vi "一体站流程自动启动.vi"(11 "参数":T1={"CODCr"={"启动测量模式"={"测量模式"=enum."水样测量"}, "确定按钮"=TRUE}, "参数启用"={"多参数"=FALSE, "CODMn"=FALSE, "总磷"=FALSE, "总氮"=FALSE, "氨氮"=FALSE, "CODcr"=FALSE}}) -> ()   [LabVIEW 2016, in "PLC.lvlib"]
uses:
  PLC.lvlib
  API/CodCr/CodCr.lvlib
panel:
  out "枚举":enum16{"初始化", "采配水启动", "等待", "配水", "排水", "结束"}(ring)
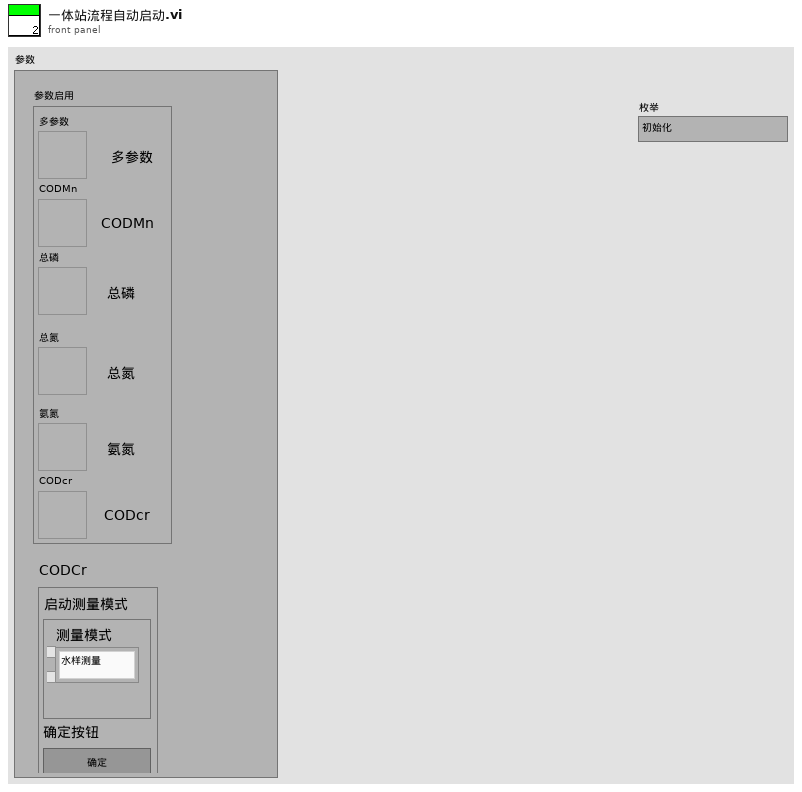
[diagram p1: front panel]
types:
  T1 = cluster{"CODCr":cluster{"启动测量模式":cluster{"测量模式":enum16{"水样测量", "标样核查", "零点核查", "跨度核查", "空白测试", "加标回收", "平行样", "校零", "校标"}}, "确定按钮":bool}, "参数启用":cluster{"多参数":bool, "CODMn":bool, "总磷":bool, "总氮":bool, "氨氮":bool, "CODcr":bool}}
  T2 = cluster{"命令":string, cluster{"starting address":u16, "holding register value":u16}}
  T3 = enum16{"待机", "启动氨氮", "氨氮测量中", "启动总磷", "总磷测量中", "结束"}
  T4 = cluster{"站号 2":u16, "量程切换":enum32{"H", "L", "AUTO"}, "控制命令":enum16{"启动测量", "标样核查", "零点核查", "跨度核查", "空白测试", "平行样测试", "加标回收", "空白校准", "标样校准", "初始化（清洗）", "停止测试", "仪器重启", "校时", "模式设置", "测量间隔设置"}, "模式设置":enum16{"待机", "连续模式", "周期模式", "定点模式", "受控模式", "手动模式"}, "测量间隔":u16}
  T5 = cluster{"测量模式":enum16{"水样测量", "标样核查", "零点核查", "跨度核查", "空白测试", "加标回收", "平行样", "校零", "校标"}}
  T6 = cluster{"时间标识":timestamp, "设备":string, "日志信息":string, "流程参数":string}
  T7 = cluster{"时间标识":timestamp, "设备":string, "日志信息":string}
  T8 = enum16{"空闲", "水样测试", "标样核查", "零点核查", "跨度核查", "空白测试", "平行样测试", "加标回收", "空白校准", "标样校准", "初始化（清洗）"}
  T9 = cluster{"R0":i16, "R1":i16, "R2":i16, "R3":i16, "R4":i16, "R5":i16, "R6":i16, "R7":i16, "R8":i16, "R9":i16, "R10":i16, "R11":i16, "R12":i16, "R13":i16, "R14":i16, "R15":i16, "R16":i16, "R17":i16, "R18":i16, "R19":i16, "R20":i16, "R21":i16, "R22":i16, "R23":i16, "R24":i16, "R25":i16, "R26":i16, "R27":i16, "R28":i16, "R29":i16, "R30":i16, "R31":i16, "R32":i16, "R33":i16, "R34":i16, "R35":i16, "R36":i16, "R37":i16, "R38":i16, "R39":i16, "R40":i16, "R41":i16, "R42":i16, "R43":i16, "R44":i16, "R45":i16, "R46":i16, "R47":i16, "R48":i16, "R49":i16, "R50":i16, "R51":i16, "R52":i16, "R53":i16, "R54":i16, "R55":i16, "R56":i16}
  T10 = enum32{"Bad", "Idle", "Run top level", "Running"}
  T11 = cluster{"水样测试量程模式":enum16{"H", "L", "AUTO"}, "空白核查量程模式":enum16{"H", "L", "AUTO"}, "跨度核查量程模式":enum16{"H", "L", "AUTO"}}
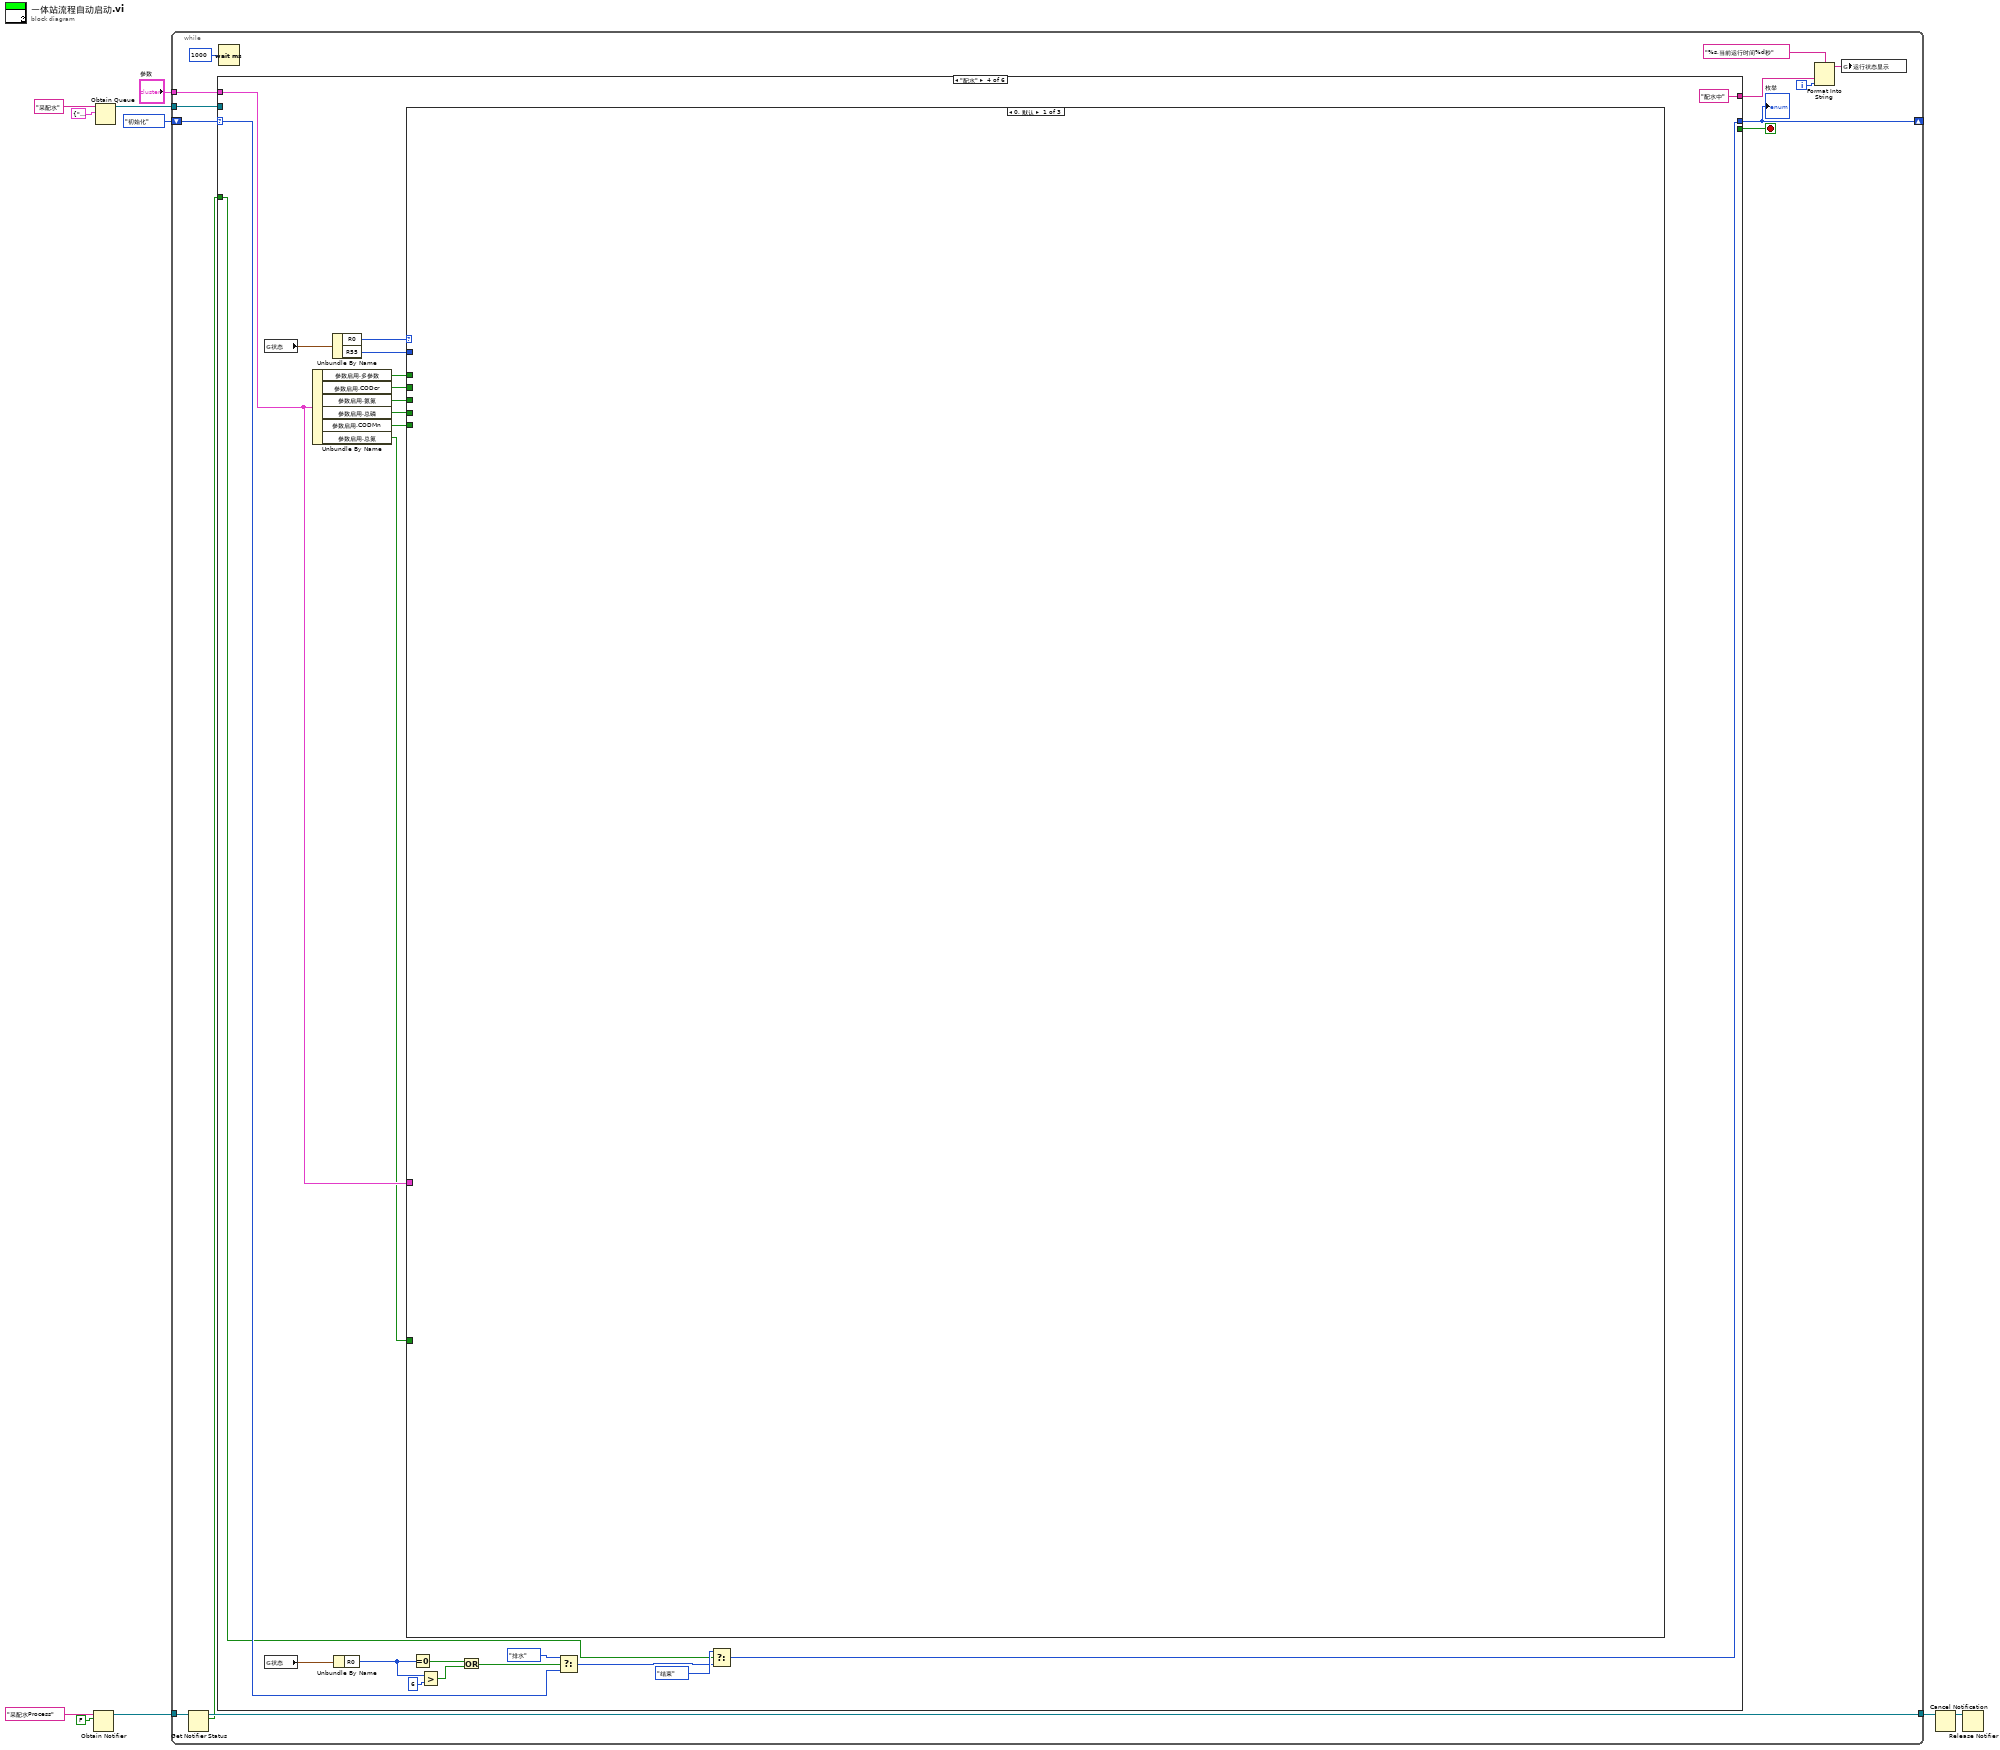
[diagram p0: block diagram]
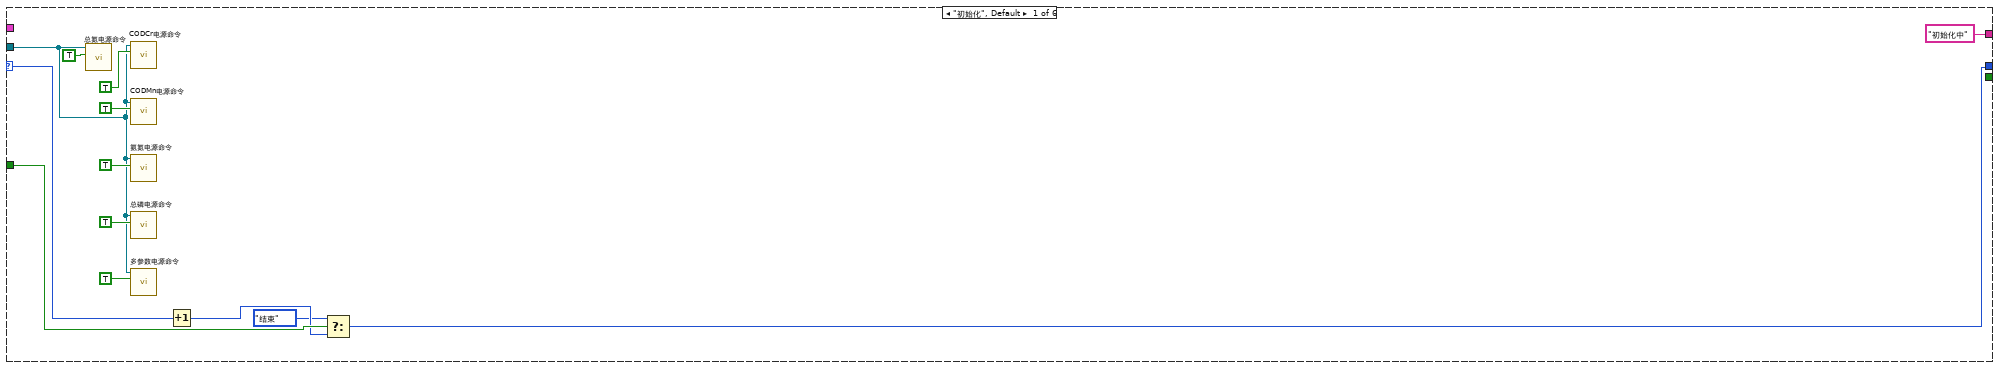
[diagram p2: hidden frame]
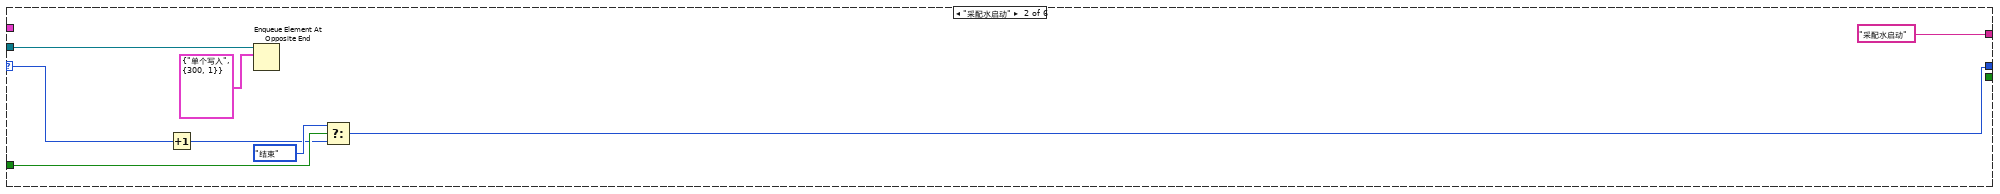
[diagram p3: hidden frame]
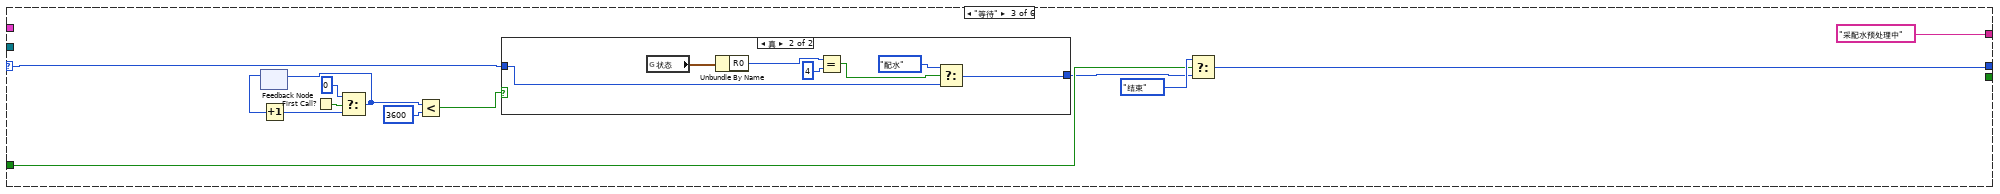
[diagram p4: hidden frame]
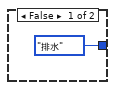
[diagram p5: hidden frame]
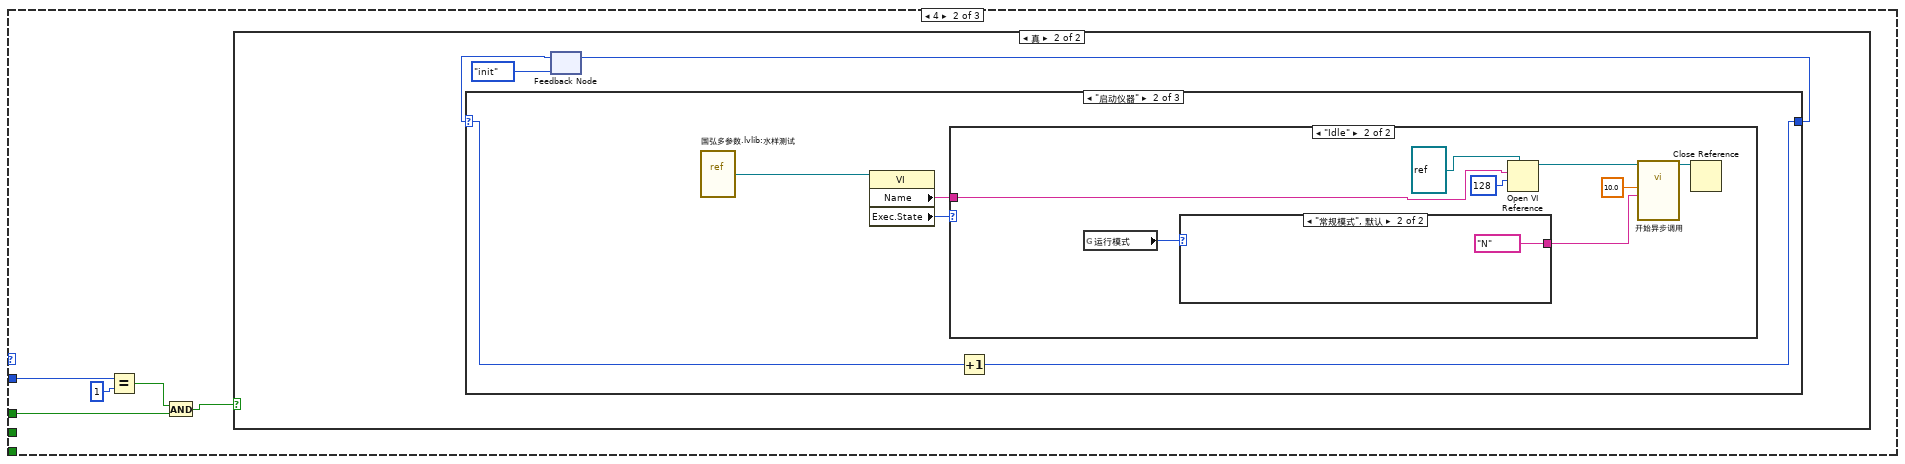
[diagram p6: hidden frame]
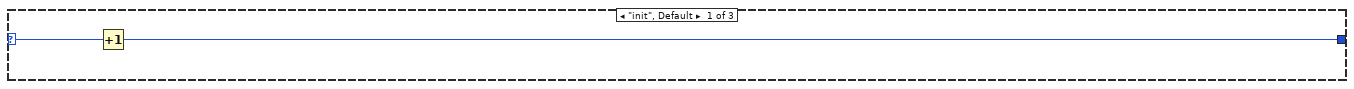
[diagram p8: hidden frame]
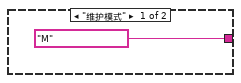
[diagram p10: hidden frame]
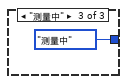
[diagram p11: hidden frame]
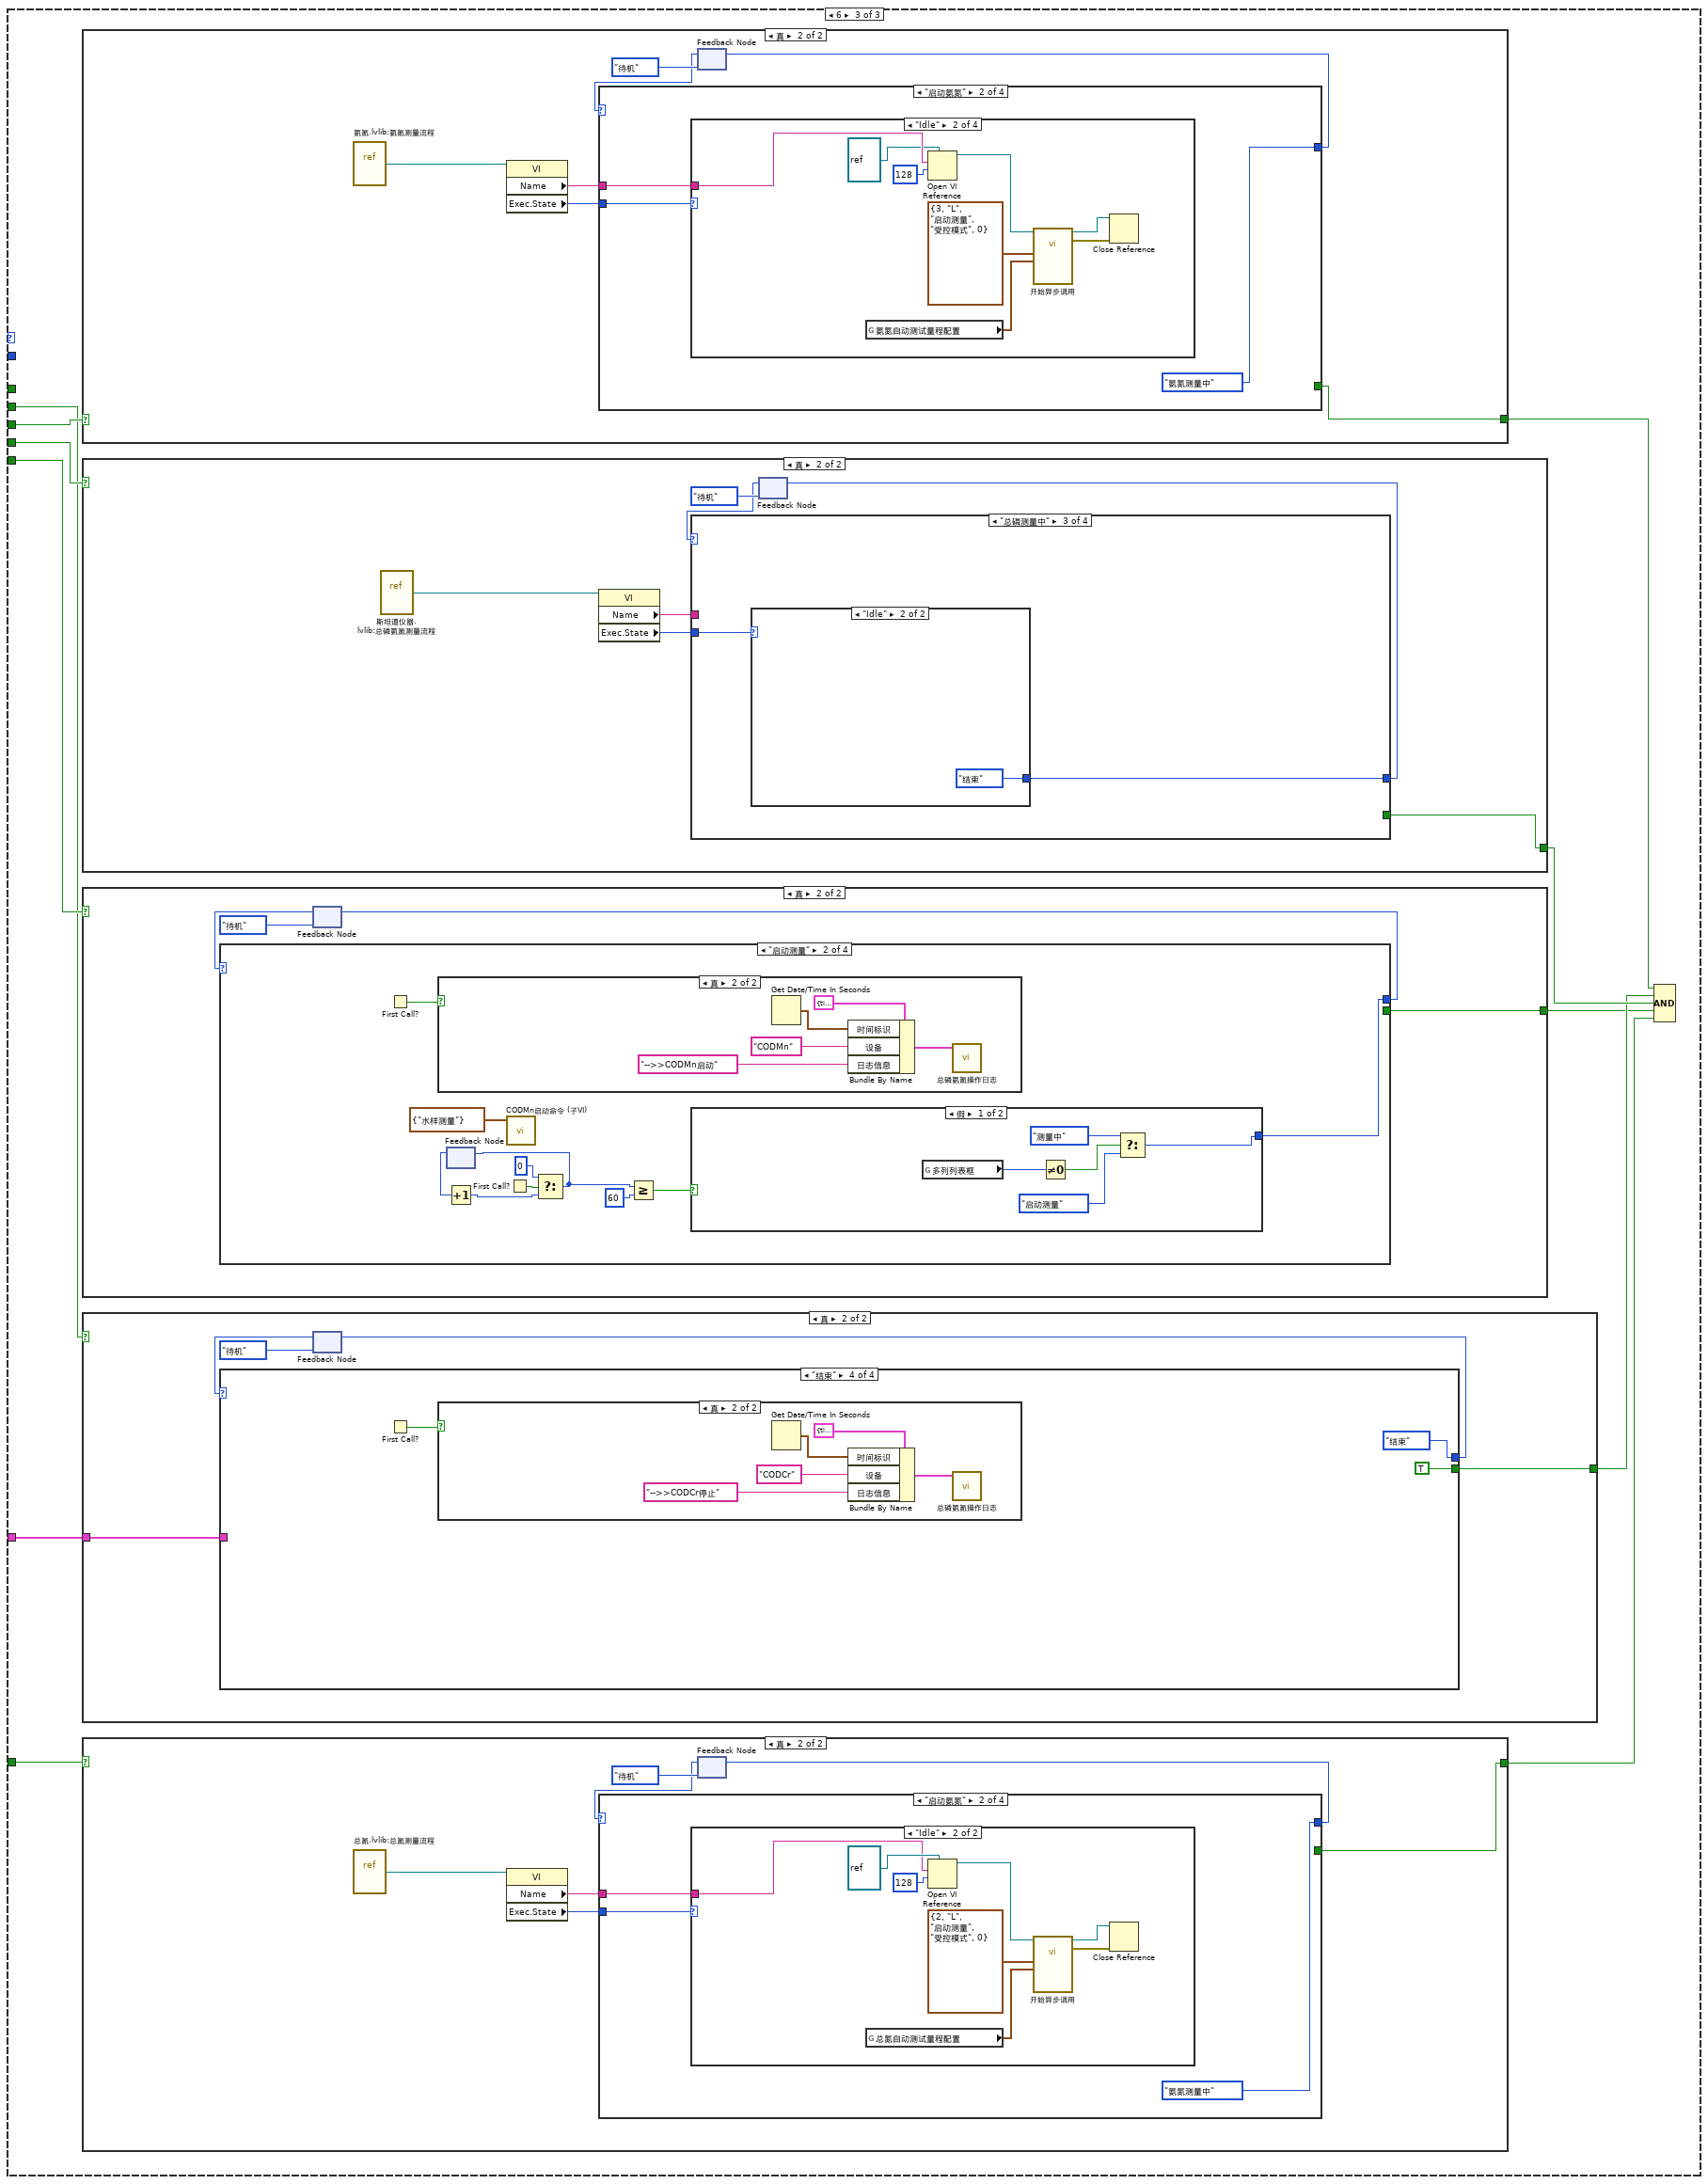
[diagram p12: hidden frame]
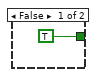
[diagram p13: hidden frame]
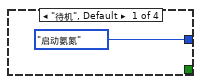
[diagram p14: hidden frame]
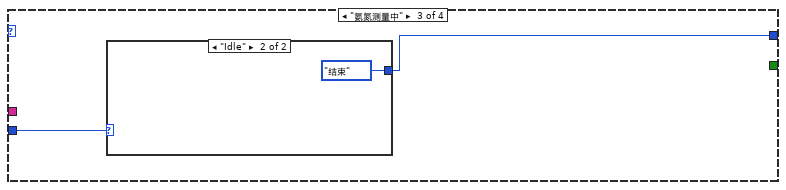
[diagram p16: hidden frame]
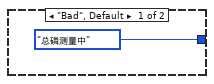
[diagram p17: hidden frame]
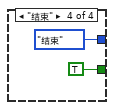
[diagram p18: hidden frame]
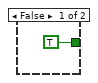
[diagram p19: hidden frame]
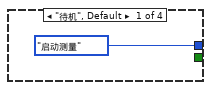
[diagram p20: hidden frame]
diagram:
  n1 = Obtain Notifier(name (unnamed)="采配水Process" ("名称（未命名）"), notification data type=FALSE) -> (notifier out=w3:refnum<notifier>)  [unwired: 2 in, 2 out]
  n2 = Obtain Queue(name (unnamed)="采配水" ("名称（未命名）"), element data type=cluster{"命令":string, "数据":variant} {"命令"="", "数据"=variant}) -> (queue out=w8:refnum<queue>)  [unwired: 3 in, 2 out]
  n3 = while {
    tunnel: w8 -> [w23]
    shift-right: [w21] -> _
    shift-left: enum16{"初始化", "采配水启动", "等待", "配水", "排水", "结束"}."初始化" ("枚举") -> [w22]
    tunnel: "参数" -> [w19]
    tunnel: w3 -> [w18]
    tunnel: [w17] -> w2
    i -> [w14]
    stop <- w13 stop-if-true
    n4 = Get Notifier Status(notifier=w18) -> (notifier out=w17:refnum<notifier>, current notification=w12:bool)  [unwired: 1 in, 3 out]
    n5 = case shown="\"配水\"" w22 {
      selector: w22 -> [w36 w42 w55 w87 w306 w312]
      tunnel: w23 -> [w25 w43 _ _ w307 _]
      tunnel: [w32 w37 w45 w83 w301 w311] -> w21
      tunnel: [_ _ _ _ _ TRUE] -> w13
      tunnel: w19 -> [_ _ _ w79 _ _]
      tunnel: ["初始化中" ("输入 1") "采配水启动" ("输入 1") "采配水预处理中" ("输入 1") "配水中" ("输入 1") "排水中" ("输入 1") "结束" ("输入 1")] -> w15
      tunnel: w12 -> [w34 w39 w47 w85 w303 _]
      frame "初始化", Default {
        n6 = call "总氮电源命令.vi"("通电/断电"=TRUE, "队列"=w25) -> ()  [unwired: 9 in, 1 out]
        n7 = call "CODCr电源命令.vi"("通电/断电"=TRUE, "队列"=w25) -> ()  [unwired: 9 in, 1 out]
        n8 = call "CODMn电源命令.vi"("通电/断电"=TRUE, "队列"=w25) -> ()  [unwired: 9 in, 1 out]
        n9 = call "氨氮电源命令.vi"("通电/断电"=TRUE, "队列"=w25) -> ()  [unwired: 9 in, 1 out]
        n10 = call "总磷电源命令.vi"("通电/断电"=TRUE, "队列"=w25) -> ()  [unwired: 9 in, 1 out]
        n11 = call "多参数电源命令.vi"("通电/断电"=TRUE, "队列"=w25) -> ()  [unwired: 9 in, 1 out]
        n12 = Increment(x=w36) -> (x+1=w33:enum16{"初始化", "采配水启动", "等待", "配水", "排水", "结束"})
        n13 = Select(t=enum16{"初始化", "采配水启动", "等待", "配水", "排水", "结束"}."结束", s=w34, f=w33) -> (s? t:f=w32:enum16{"初始化", "采配水启动", "等待", "配水", "排水", "结束"})
      }
      frame "采配水启动" {
        n14 = Increment(x=w42) -> (x+1=w38:enum16{"初始化", "采配水启动", "等待", "配水", "排水", "结束"})
        n15 = Enqueue Element At Opposite End(queue=w43, element=T2 {"命令"="单个写入", {"starting address"=300, "holding register value"=1}} ("元素")) -> ()  [unwired: 2 in, 3 out]
        n16 = Select(t=enum16{"初始化", "采配水启动", "等待", "配水", "排水", "结束"}."结束", s=w39, f=w38) -> (s? t:f=w37:enum16{"初始化", "采配水启动", "等待", "配水", "排水", "结束"})
      }
      frame "等待" {
        n17 = feedback #1() -> (w52:i32)  [unwired: 1 in]
        n18 = Increment(x=w52) -> (x+1=w51:i32)
        n19 = First Call?() -> (First Call?: T/F=w53:bool)
        n20 = Select(t=0, s=w53, f=w51) -> (s? t:f=w50:i32)
        n21 = feedback-in #1(w50) -> ()
        n22 = Less?(x=w50, y=3600) -> (x < y?=w56:bool)
        n23 = case shown="真" w56 {
          tunnel: w55 -> [_ w60]
          tunnel: [enum16{"初始化", "采配水启动", "等待", "配水", "排水", "结束"}."排水" ("枚举") w59] -> w46
          frame False {
          }
          frame True {
            n24 = global read "采配水全局变量.vi" "状态"() -> (w65:T9)
            n25 = Unbundle By Name(w65) -> ("R0"=w64:i16)
            n26 = Equal?(x=w64, y=i16 4) -> (x = y?=w62:bool)
            n27 = Select(t=enum16{"初始化", "采配水启动", "等待", "配水", "排水", "结束"}."配水" ("枚举"), s=w62, f=w60) -> (s? t:f=w59:enum16{"初始化", "采配水启动", "等待", "配水", "排水", "结束"})
          }
        }
        n28 = Select(t=enum16{"初始化", "采配水启动", "等待", "配水", "排水", "结束"}."结束", s=w47, f=w46) -> (s? t:f=w45:enum16{"初始化", "采配水启动", "等待", "配水", "排水", "结束"})
      }
      frame "配水" {
        n29 = global read "采配水全局变量.vi" "状态"() -> (w70:T9)
        n30 = global read "采配水全局变量.vi" "状态"() -> (w77:T9)
        n31 = Unbundle By Name(w79) -> ("参数启用.多参数"=w68:bool, "参数启用.CODcr"=w78:bool, "参数启用.氨氮"=w82:bool, "参数启用.总磷"=w81:bool, "参数启用.CODMn"=w80:bool, "参数启用.总氮"=w71:bool)
        n32 = Unbundle By Name(w70) -> ("R0"=w69:i16, "R55"=w66:i16)
        n33 = Unbundle By Name(w77) -> ("R0"=w76:i16)
        n34 = case shown="0, 默认" w69 {
          tunnel: w82 -> [_ _ w125]
          tunnel: w81 -> [_ _ w124]
          tunnel: w80 -> [_ _ w121]
          tunnel: w79 -> [_ _ w120]
          tunnel: w78 -> [_ _ w119]
          tunnel: w71 -> [_ _ w116]
          tunnel: w68 -> [_ w90 _]
          tunnel: w66 -> [_ w93 _]
          frame 0, Default {
          }
          frame 4 {
            n35 = Equal?(x=w93, y=i16 1) -> (x = y?=w91:bool)
            n36 = And(x=w91, y=w90) -> (x .and. y?=w89:bool)
            n37 = case shown="真" w89 {
              frame False {
              }
              frame True {
                n38 = feedback #2(enum16{"init", "启动仪器", "测量中"}."init") -> (w95:enum16{"init", "启动仪器", "测量中"})
                n39 = case shown="\"启动仪器\"" w95 {
                  selector: w95 -> [w98 w103 _]
                  tunnel: [w97 w102 enum16{"init", "启动仪器", "测量中"}."测量中"] -> w96
                  frame "init", Default {
                    n40 = Increment(x=w98) -> (x+1=w97:enum16{"init", "启动仪器", "测量中"})
                  }
                  frame "启动仪器" {
                    n41 = vi-ref "国弘多参数.lvlib:水样测试.vi"() -> (w100:refnum<vi>)
                    n42 = property class="VI"(reference=w100) -> ("Name"=w99:string, "Exec.State"=w101:T10)  [unwired: 1 in, 2 out]
                    n43 = case shown="\"Idle\"" w101 {
                      tunnel: w99 -> [_ w110]
                      frame "Bad", Default {
                      }
                      frame "Idle" {
                        n44 = global read "系统变量.vi" "运行模式"() -> (w107:enum16{"维护模式", "常规模式", "应急模式", "质控模式"})
                        n45 = case shown="\"常规模式\", 默认" w107 {
                          tunnel: ["M" ("数据标记表") "N" ("数据标记表")] -> w105
                          frame "维护模式" {
                          }
                          frame "常规模式", Default {
                          }
                        }
                        n46 = Open VI Reference(type specifier VI Refnum (for type only)=refnum<vi> refnum, vi path=w110, options=128 ("选项")) -> (vi reference=w109:refnum<vi>)  [unwired: 3 in, 1 out]
                        n47 = call-by-ref "开始异步调用"(reference=w109, "数据标记表"=w105, "水样测试时间"=10.0) -> (reference out=w108:refnum<vi>)  [unwired: 11 in, 1 out]
                        n48 = Close Reference(reference=w108) -> ()  [unwired: 1 in, 1 out]
                      }
                    }
                    n49 = Increment(x=w103) -> (x+1=w102:enum16{"init", "启动仪器", "测量中"})
                  }
                  frame "测量中" {
                  }
                }
                n50 = feedback-in #2(w96) -> ()
              }
            }
          }
          frame 6 {
            n51 = case shown="真" w125 {
              tunnel: [TRUE w279] -> w123
              frame False {
              }
              frame True {
                n52 = vi-ref "氨氮.lvlib:氨氮测量流程.vi"() -> (w278:refnum<vi>)
                n53 = property class="VI"(reference=w278) -> ("Name"=w277:string, "Exec.State"=w276:T10)  [unwired: 1 in, 2 out]
                n54 = feedback #3(T3."待机") -> (w281:T3)
                n55 = case shown="\"启动氨氮\"" w281 {
                  tunnel: [T3."启动氨氮" T3."氨氮测量中" w295 T3."结束"] -> w280
                  tunnel: [_ _ _ TRUE] -> w279
                  tunnel: w277 -> [_ w285 _ _]
                  tunnel: w276 -> [_ w284 w296 _]
                  frame "待机", Default {
                  }
                  frame "启动氨氮" {
                    n56 = case shown="\"Idle\"" w284 {
                      tunnel: w285 -> [_ w291 _ _]
                      frame "Bad", Default {
                      }
                      frame "Idle" {
                        n57 = global read "系统设置全局变量.vi" "氨氮自动测试量程配置"() -> (w288:T11)
                        n58 = Open VI Reference(type specifier VI Refnum (for type only)=refnum<vi> refnum, vi path=w291, options=128 ("选项")) -> (vi reference=w292:refnum<vi>)  [unwired: 3 in, 1 out]
                        n59 = call-by-ref "开始异步调用"(reference=w292, "量程模式"=w288, "参数"=T4 {"站号 2"=3, "量程切换"=enum."L", "控制命令"=enum."启动测量", "模式设置"=enum."受控模式", "测量间隔"=0}) -> (reference out=w293:refnum<vi>, error out=w294:errorcluster)  [unwired: 11 in]
                        n60 = Close Reference(reference=w293, error in (no error)=w294) -> ()  [unwired: 1 out]
                      }
                      frame "Run top level" {
                      }
                      frame "Running" {
                      }
                    }
                  }
                  frame "氨氮测量中" {
                    n61 = case shown="\"Bad\", 默认" w296 {
                      tunnel: [T3."氨氮测量中" T3."结束"] -> w295
                      frame "Bad", Default {
                      }
                      frame "Idle" {
                      }
                    }
                  }
                  frame "结束" {
                  }
                }
                n62 = feedback-in #3(w280) -> ()
              }
            }
            n63 = case shown="真" w124 {
              tunnel: [TRUE w253] -> w122
              frame False {
              }
              frame True {
                n64 = vi-ref "斯坦道仪器.lvlib:总磷氨氮测量流程.vi"() -> (w252:refnum<vi>)
                n65 = property class="VI"(reference=w252) -> ("Name"=w251:string, "Exec.State"=w250:T10)  [unwired: 1 in, 2 out]
                n66 = feedback #4(T3."待机") -> (w255:T3)
                n67 = case shown="\"总磷测量中\"" w255 {
                  tunnel: [T3."启动总磷" T3."总磷测量中" w269 T3."结束"] -> w254
                  tunnel: [_ _ _ TRUE] -> w253
                  tunnel: w251 -> [_ w260 _ _]
                  tunnel: w250 -> [_ w259 w270 _]
                  frame "待机", Default {
                  }
                  frame "启动总磷" {
                    n68 = case shown="\"Idle\"" w259 {
                      tunnel: w260 -> [_ w267]
                      frame "Bad", Default {
                      }
                      frame "Idle" {
                        n69 = global read "系统设置全局变量.vi" "总磷自动测试量程配置"() -> (w262:T11)
                        n70 = Open VI Reference(type specifier VI Refnum (for type only)=refnum<vi> refnum, vi path=w267, options=128 ("选项")) -> (vi reference=w266:refnum<vi>)  [unwired: 3 in, 1 out]
                        n71 = call-by-ref "开始异步调用"(reference=w266, "量程模式"=w262, "参数"=T4 {"站号 2"=1, "量程切换"=enum."L", "控制命令"=enum."启动测量", "模式设置"=enum."受控模式", "测量间隔"=0}) -> (reference out=w265:refnum<vi>, error out=w264:errorcluster)  [unwired: 11 in]
                        n72 = Close Reference(reference=w265, error in (no error)=w264) -> ()  [unwired: 1 out]
                      }
                    }
                  }
                  frame "总磷测量中" {
                    n73 = case shown="\"Idle\"" w270 {
                      tunnel: [T3."总磷测量中" T3."结束"] -> w269
                      frame "Bad", Default {
                      }
                      frame "Idle" {
                      }
                    }
                  }
                  frame "结束" {
                  }
                }
                n74 = feedback-in #4(w254) -> ()
              }
            }
            n75 = case shown="真" w121 {
              tunnel: [TRUE w153] -> w117
              frame False {
              }
              frame True {
                n76 = feedback #5(enum16{"待机", "启动测量", "测量中", "结束"}."待机") -> (w155:enum16{"待机", "启动测量", "测量中", "结束"})
                n77 = case shown="\"启动测量\"" w155 {
                  tunnel: [enum16{"待机", "启动测量", "测量中", "结束"}."启动测量" w167 w186 enum16{"待机", "启动测量", "测量中", "结束"}."结束"] -> w154
                  tunnel: [_ _ _ TRUE] -> w153
                  frame "待机", Default {
                  }
                  frame "启动测量" {
                    n78 = First Call?() -> (First Call?: T/F=w158:bool)
                    n79 = case shown="真" w158 {
                      frame False {
                      }
                      frame True {
                        n80 = Get Date/Time In Seconds() -> (seconds since 1Jan1904=w172:timestamp)
                        n81 = Bundle By Name(cluster=T6 {"时间标识"=timestamp(0 s since 1904-01-01), "设备"="", "日志信息"="", "流程参数"=""} ("data in"), "时间标识"=w172, "设备"="CODMn", "日志信息"="-->>CODMn启动") -> (w168:T6)
                        n82 = call "总磷氨氮操作日志.vi"("data in"=w168) -> ()  [unwired: 11 in]
                      }
                    }
                    n83 = feedback #6() -> (w163:i32)  [unwired: 1 in]
                    n84 = Increment(x=w163) -> (x+1=w164:i32)
                    n85 = First Call?() -> (First Call?: T/F=w162:bool)
                    n86 = call "CODMn启动命令 (子VI).vi"("启动测量模式"=T5 {"测量模式"=enum."水样测量"}) -> ()  [unwired: 11 in]
                    n87 = Select(t=0, s=w162, f=w164) -> (s? t:f=w165:i32)
                    n88 = feedback-in #6(w165) -> ()
                    n89 = Greater Or Equal?(x=w165, y=60) -> (x >= y?=w160:bool)
                    n90 = case shown="假" w160 {
                      tunnel: [w174 enum16{"待机", "启动测量", "测量中", "结束"}."结束"] -> w167
                      frame False {
                        n91 = global read "运行时序全局变量.vi" "多列列表框"() -> (w173:i32)
                        n92 = Not Equal To 0?(x=w173) -> (x != 0?=w175:bool)
                        n93 = Select(t=enum16{"待机", "启动测量", "测量中", "结束"}."测量中", s=w175, f=enum16{"待机", "启动测量", "测量中", "结束"}."启动测量") -> (s? t:f=w174:enum16{"待机", "启动测量", "测量中", "结束"})
                      }
                      frame True {
                        n94 = Get Date/Time In Seconds() -> (seconds since 1Jan1904=w178:timestamp)
                        n95 = Bundle By Name(cluster=T7 {"时间标识"=timestamp(0 s since 1904-01-01), "设备"="", "日志信息"=""} ("data in"), "时间标识"=w178, "设备"="CODMn", "日志信息"="CODMn启动失败") -> (w182:T7)
                        n96 = call "总磷氨氮报警信息.vi"("data in"=w182) -> ()  [unwired: 11 in]
                      }
                    }
                  }
                  frame "测量中" {
                    n97 = global read "运行时序全局变量.vi" "多列列表框"() -> (w185:i32)
                    n98 = Equal To 0?(x=w185) -> (x = 0?=w184:bool)
                    n99 = case shown="假" w184 {
                      tunnel: [w187 enum16{"待机", "启动测量", "测量中", "结束"}."结束"] -> w186
                      frame False {
                        n100 = flat-sequence {
                          tunnel: [enum16{"待机", "启动测量", "测量中", "结束"}."测量中"] -> w187
                          frame #0 {
                            n101 = Wait (ms)(milliseconds to wait=u32 1000 ("等待时间（毫秒）")) -> ()  [unwired: 1 out]
                          }
                          frame #1 {
                          }
                        }
                      }
                      frame True {
                      }
                    }
                  }
                  frame "结束" {
                    n102 = First Call?() -> (First Call?: T/F=w191:bool)
                    n103 = case shown="真" w191 {
                      frame False {
                      }
                      frame True {
                        n104 = Get Date/Time In Seconds() -> (seconds since 1Jan1904=w198:timestamp)
                        n105 = Bundle By Name(cluster=T6 {"时间标识"=timestamp(0 s since 1904-01-01), "设备"="", "日志信息"="", "流程参数"=""} ("data in"), "时间标识"=w198, "设备"="CODMn", "日志信息"="-->>CODMn停止") -> (w194:T6)
                        n106 = call "总磷氨氮操作日志.vi"("data in"=w194) -> ()  [unwired: 11 in]
                      }
                    }
                  }
                }
                n107 = feedback-in #5(w154) -> ()
              }
            }
            n108 = case shown="真" w119 {
              tunnel: [TRUE w201] -> w118
              tunnel: w120 -> [_ w200]
              frame False {
              }
              frame True {
                n109 = feedback #7(enum16{"待机", "启动测量", "测量中", "结束"}."待机") -> (w203:enum16{"待机", "启动测量", "测量中", "结束"})
                n110 = case shown="\"结束\"" w203 {
                  tunnel: [enum16{"待机", "启动测量", "测量中", "结束"}."启动测量" w215 w236 enum16{"待机", "启动测量", "测量中", "结束"}."结束"] -> w202
                  tunnel: w200 -> [_ w216 _ _]
                  tunnel: [_ _ _ TRUE] -> w201
                  frame "待机", Default {
                  }
                  frame "启动测量" {
                    n111 = Unbundle By Name(w216) -> ("CODCr.启动测量模式"=w214:T5)
                    n112 = First Call?() -> (First Call?: T/F=w206:bool)
                    n113 = case shown="真" w206 {
                      frame False {
                      }
                      frame True {
                        n114 = Get Date/Time In Seconds() -> (seconds since 1Jan1904=w221:timestamp)
                        n115 = Bundle By Name(cluster=T6 {"时间标识"=timestamp(0 s since 1904-01-01), "设备"="", "日志信息"="", "流程参数"=""} ("data in"), "时间标识"=w221, "设备"="CODCr", "日志信息"="-->>CODCr启动") -> (w217:T6)
                        n116 = call "总磷氨氮操作日志.vi"("data in"=w217) -> ()  [unwired: 11 in]
                      }
                    }
                    n117 = call "CODCr启动命令 (子VI).vi"("启动测量模式"=w214) -> ()  [unwired: 11 in]
                    n118 = feedback #8() -> (w210:i32)  [unwired: 1 in]
                    n119 = Increment(x=w210) -> (x+1=w211:i32)
                    n120 = First Call?() -> (First Call?: T/F=w209:bool)
                    n121 = Select(t=0, s=w209, f=w211) -> (s? t:f=w212:i32)
                    n122 = feedback-in #8(w212) -> ()
                    n123 = Greater Or Equal?(x=w212, y=60) -> (x >= y?=w207:bool)
                    n124 = case shown="真" w207 {
                      tunnel: [w222 enum16{"待机", "启动测量", "测量中", "结束"}."结束"] -> w215
                      frame False {
                        n125 = global read "CODCr工作状态.vi" "工作状态"() -> (w223:T8)
                        n126 = Not Equal To 0?(x=w223) -> (x != 0?=w224:bool)
                        n127 = Select(t=enum16{"待机", "启动测量", "测量中", "结束"}."测量中", s=w224, f=enum16{"待机", "启动测量", "测量中", "结束"}."启动测量") -> (s? t:f=w222:enum16{"待机", "启动测量", "测量中", "结束"})
                      }
                      frame True {
                        n128 = Get Date/Time In Seconds() -> (seconds since 1Jan1904=w227:timestamp)
                        n129 = Bundle By Name(cluster=T7 {"时间标识"=timestamp(0 s since 1904-01-01), "设备"="", "日志信息"=""} ("data in"), "时间标识"=w227, "设备"="CODCr", "日志信息"="CODCr启动失败") -> (w231:T7)
                        n130 = call "总磷氨氮报警信息.vi"("data in"=w231) -> ()  [unwired: 11 in]
                      }
                    }
                  }
                  frame "测量中" {
                    n131 = global read "CODCr工作状态.vi" "工作状态"() -> (w235:T8)
                    n132 = Equal?(x=w235, y=T8."空闲" ("工作状态")) -> (x = y?=w234:bool)
                    n133 = case shown="假" w234 {
                      tunnel: [w237 enum16{"待机", "启动测量", "测量中", "结束"}."结束"] -> w236
                      frame False {
                        n134 = flat-sequence {
                          tunnel: [enum16{"待机", "启动测量", "测量中", "结束"}."测量中"] -> w237
                          frame #0 {
                            n135 = Wait (ms)(milliseconds to wait=u32 1000 ("等待时间（毫秒）")) -> ()  [unwired: 1 out]
                          }
                          frame #1 {
                          }
                        }
                      }
                      frame True {
                      }
                    }
                  }
                  frame "结束" {
                    n136 = First Call?() -> (First Call?: T/F=w241:bool)
                    n137 = case shown="真" w241 {
                      frame False {
                      }
                      frame True {
                        n138 = Get Date/Time In Seconds() -> (seconds since 1Jan1904=w248:timestamp)
                        n139 = Bundle By Name(cluster=T6 {"时间标识"=timestamp(0 s since 1904-01-01), "设备"="", "日志信息"="", "流程参数"=""} ("data in"), "时间标识"=w248, "设备"="CODCr", "日志信息"="-->>CODCr停止") -> (w244:T6)
                        n140 = call "总磷氨氮操作日志.vi"("data in"=w244) -> ()  [unwired: 11 in]
                      }
                    }
                  }
                }
                n141 = feedback-in #7(w202) -> ()
              }
            }
            n142 = case shown="真" w116 {
              tunnel: [TRUE w130] -> w115
              frame False {
              }
              frame True {
                n143 = vi-ref "总氮.lvlib:总氮测量流程.vi"() -> (w129:refnum<vi>)
                n144 = property class="VI"(reference=w129) -> ("Name"=w128:string, "Exec.State"=w127:T10)  [unwired: 1 in, 2 out]
                n145 = feedback #9(T3."待机") -> (w132:T3)
                n146 = case shown="\"启动氨氮\"" w132 {
                  tunnel: [T3."启动氨氮" T3."氨氮测量中" w146 T3."结束"] -> w131
                  tunnel: [_ _ _ TRUE] -> w130
                  tunnel: w128 -> [_ w137 _ _]
                  tunnel: w127 -> [_ w136 w147 _]
                  frame "待机", Default {
                  }
                  frame "启动氨氮" {
                    n147 = case shown="\"Idle\"" w136 {
                      tunnel: w137 -> [_ w138]
                      frame "Bad", Default {
                      }
                      frame "Idle" {
                        n148 = global read "系统设置全局变量.vi" "总氮自动测试量程配置"() -> (w140:T11)
                        n149 = Open VI Reference(type specifier VI Refnum (for type only)=refnum<vi> refnum, vi path=w138, options=128 ("选项")) -> (vi reference=w144:refnum<vi>)  [unwired: 3 in, 1 out]
                        n150 = call-by-ref "开始异步调用"(reference=w144, "量程模式"=w140, "参数"=T4 {"站号 2"=2, "量程切换"=enum."L", "控制命令"=enum."启动测量", "模式设置"=enum."受控模式", "测量间隔"=0}) -> (reference out=w143:refnum<vi>, error out=w142:errorcluster)  [unwired: 11 in]
                        n151 = Close Reference(reference=w143, error in (no error)=w142) -> ()  [unwired: 1 out]
                      }
                    }
                  }
                  frame "氨氮测量中" {
                    n152 = case shown="\"Idle\"" w147 {
                      tunnel: [T3."总磷测量中" T3."结束"] -> w146
                      frame "Bad", Default {
                      }
                      frame "Idle" {
                      }
                    }
                  }
                  frame "结束" {
                  }
                }
                n153 = feedback-in #9(w131) -> ()
              }
            }
            n154 = Compound Arithmetic op=AND ("复合运算")(w123, w118, w122, w117, w115) -> ()  [unwired: 1 out]
          }
        }
        n155 = Equal To 0?(x=w76) -> (x = 0?=w73:bool)
        n156 = Greater?(x=w76, y=i16 6) -> (0:w74:bool)
        n157 = Or(x=w73, y=w74) -> (x .or. y?=w72:bool)
        n158 = Select(t=enum16{"初始化", "采配水启动", "等待", "配水", "排水", "结束"}."排水" ("枚举"), s=w72, f=w87) -> (s? t:f=w84:enum16{"初始化", "采配水启动", "等待", "配水", "排水", "结束"})
        n159 = Select(t=enum16{"初始化", "采配水启动", "等待", "配水", "排水", "结束"}."结束", s=w85, f=w84) -> (s? t:f=w83:enum16{"初始化", "采配水启动", "等待", "配水", "排水", "结束"})
      }
      frame "排水" {
        n160 = Increment(x=w306) -> (x+1=w302:enum16{"初始化", "采配水启动", "等待", "配水", "排水", "结束"})
        n161 = Enqueue Element At Opposite End(queue=w307, element=T2 {"命令"="单个写入", {"starting address"=303, "holding register value"=1}} ("元素")) -> ()  [unwired: 2 in, 3 out]
        n162 = Select(t=enum16{"初始化", "采配水启动", "等待", "配水", "排水", "结束"}."结束", s=w303, f=w302) -> (s? t:f=w301:enum16{"初始化", "采配水启动", "等待", "配水", "排水", "结束"})
      }
      frame "结束" {
        n163 = Increment(x=w312) -> (x+1=w311:enum16{"初始化", "采配水启动", "等待", "配水", "排水", "结束"})
      }
    }
    "枚举" <- w21
    n164 = Wait (ms)(milliseconds to wait=u32 1000 ("等待时间（毫秒）")) -> ()  [unwired: 1 out]
    n165 = Format Into String(format string="%s,当前运行时间%d秒" ("格式字符串"), w15, w14) -> (resulting string=w11:string)  [unwired: 2 in, 1 out]
    n166 = global write "采配水全局变量.vi" "运行状态显示"(w11) -> ()
  }
  n167 = Cancel Notification(0:w2) -> (8:w1:refnum<notifier>)  [unwired: 1 in, 2 out]
  n168 = Release Notifier(notifier=w1) -> ()  [unwired: 2 in, 3 out]
